vi "Periodic Tasks.vi"(8 "error in (no error)":errorcluster) -> ()   [LabVIEW 2014]
doc: "This VI runs in parallel to other tasks. It can contain as many user-defined periodic loops as you need. These can carry out PID or other sorts of timed response."
uses:
  <vilib>/Rock Robotics/WPI/Joystick/WPI_JoystickGetSetRefNum.vi
  <vilib>/Rock Robotics/WPI/RobotDrive/WPI_RobotDriveGetSetRefNum.vi
panel:
  in  "InputSelect":enum16{"RGB", "ColorBox"}(ring)=enum."ColorBox"
  in  "Position Speed":u32(slide)=20 scale=0.0..200.0
  out "B":u8
  out "G":u8=200
  out "R":u8=39
  out "Resolved Color":u32=2607104 format="%.0x"
  in  "Color Box":u32(colorbox)=12451697
  in  "LED Position":u8(slide)=7 scale=0.0..30.0
  in  "Brightness":u8(slide)=255 scale=0.0..255.0
  out "error out":errorcluster
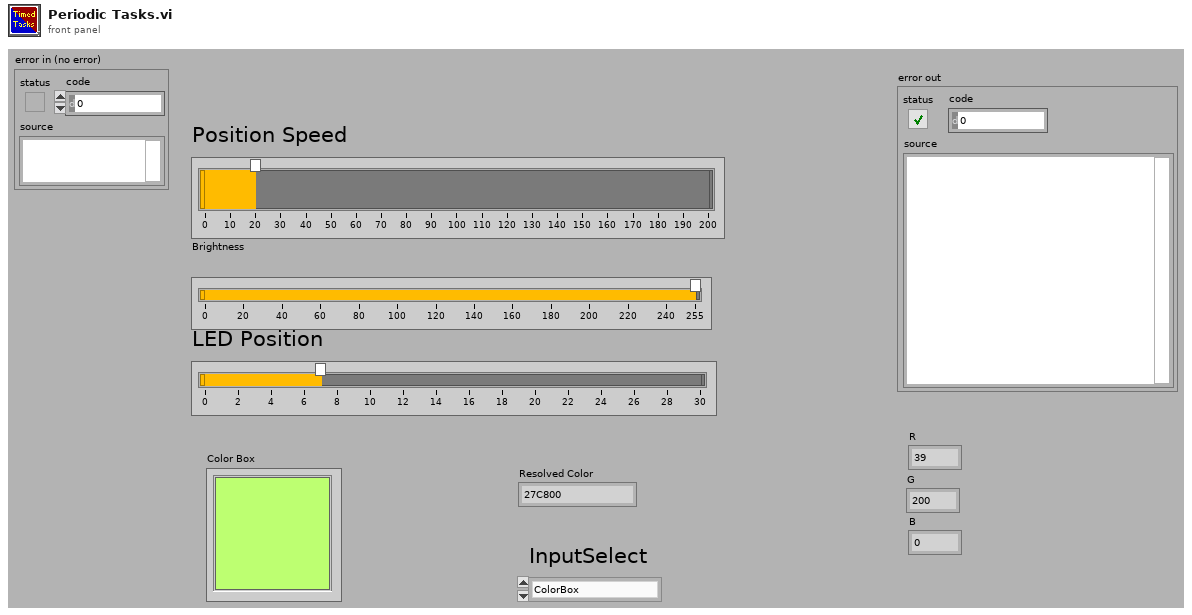
[diagram p1: front panel]
types:
  T1 = typedef "WPI_JoystickDevRef.ctl" = cluster{"Device":T2}
  T2 = typedef "WPI_JoystickDeviceEnum.ctl" = enum16{"USB 0", "USB 1", "USB 2", "USB 3", "USB 4", "USB 5"}
  T3 = typedef "WPI_RobotDriveDevRef.ctl" = cluster{"DevStatus":errorcluster, "Motors[]":T4[], "Square Inputs":bool, "Max Output":dbl}
  T4 = typedef "WPI_MotorControlDeviceRef.ctl" = cluster{"DeviceStatus":errorcluster, "Type":T5, "PWM":cluster{"Controller":T6, "PWM Channel":T7, "DeadBand":T8}, "CAN":cluster{"Device Number":u8, "Control Mode":T9, "Semaphore":T10, "Max Vout":dbl, "TalonSRX Control Mode":T11}, "Invert":bool, "TransformRef":T12, "InvTransformRef":T12}
  T5 = typedef "WPI_MotorControlType.ctl" = enum16{"PWM", "CAN", "CANTalonSRX"}
  T6 = typedef "FPGA_TypedefDigitalModule.ctl" = enum16{"Controller 1"}
  T7 = typedef "FPGA_DIOPWMChannel.ctl" = enum8{"PWM 0", "PWM 1", "PWM 2", "PWM 3", "PWM 4", "PWM 5", "PWM 6", "PWM 7", "PWM 8", "PWM 9", "PWM MXP 0", "PWM MXP 1", "PWM MXP 2", "PWM MXP 3", "PWM MXP 4", "PWM MXP 5", "PWM MXP 6", "PWM MXP 7", "PWM MXP 8", "PWM MXP 9", "Invalid"}
  T8 = typedef "WPI_PWMDeadband.ctl" = cluster{"Name":string, "maxPositivePwm":i32, "minPositivePwm":i32, "centerPwm":i32, "maxNegativePwm":i32, "minNegativePwm":i32, "angularRange":u16}
  T9 = typedef "WPI_CANJaguar_ControlMode.ctl" = enum8{"Percent VBus", "Current", "Speed", "Position", "Voltage"}
  T10 = typedef "Semaphore RefNum" = refnum<k1>
  T11 = typedef "WPI_CANTalonSRX_APIControlMode.ctl" = enum8{"Percent VBus", "Speed", "Position", "Slave", "Unchanged / Invalid"}
  T12 = typedef "WPI_PWMTransform_ConPane.ctl" = refnum<vi>
  T13 = cluster{"JoystickDevRef":T1, "RobotDriveDevRef":T3}
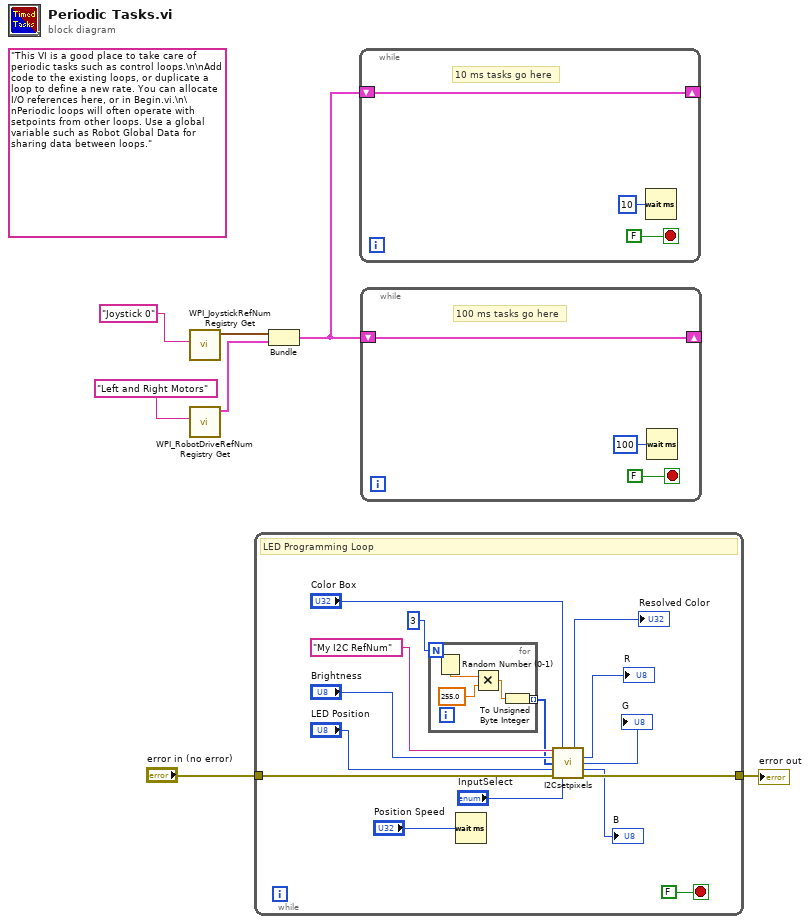
[diagram p0: block diagram]
diagram:
  (unwired) "This VI is a good place to take care of periodic tasks such as control loops.\n\nAdd code to the existing loops, or duplicate a loop to define a new rate. You can allocate I/O references here, or in Begin.vi.\n\nPeriodic loops will often operate with setpoints from other loops. Use a global variable such as Robot Global Data for sharing data between loops."
  n1 = call <vilib>:"WPI_JoystickRefNum Registry Get.vi"("refnum name"="Joystick 0") -> ("JoystickDevRef"=w5:T1)  [unwired: 1 in, 9 out]
  n2 = call <vilib>:"WPI_RobotDriveRefNum Registry Get.vi"("refnum name"="Left and Right Motors") -> ("RobotDriveDevRef"=w4:T3)  [unwired: 1 in, 9 out]
  n3 = while {
    tunnel: "error in (no error)" -> [w21]
    tunnel: [w20] -> w1
    stop <- FALSE stop-if-true
    # "LED Programming Loop"
    n4 = for {
      N: 3 -> [_]
      tunnel: [w23] -> w9 mode=indexing
      n5 = Random Number (0-1)() -> (number: 0 to 1=w25:dbl)
      n6 = Multiply(x=w25, y=255.0) -> (x*y=w24:dbl)
      n7 = To Unsigned Byte Integer(number=w24) -> (unsigned 8bit integer=w23:u8)
    }
    n8 = Wait (ms)(milliseconds to wait="Position Speed") -> ()  [unwired: 1 out]
    n9 = call "I2Csetpixels.vi"("I2C Reference In"="My I2C RefNum" ("refnum name"), "Color Box"="Color Box", "Brightness (0-255)"="Brightness", "RGB Array"=w9, "LED Position"="LED Position", "Error In"=w21, "InputSelect"="InputSelect") -> ("Resolved Color"=→"Resolved Color":u32, "R"=→"R":u8, "G"=→"G":u8, "B"=→"B":u8, "Error Out"=w20:errorcluster)  [unwired: 3 in, 1 out]
  }
  "error out" <- w1
  n10 = Bundle("JoystickDevRef"=w5, "RobotDriveDevRef"=w4) -> (w3:T13)  [unwired: 1 out]
  n11 = while {
    shift-right: [w27] -> _
    shift-left: w3 -> [w27]
    stop <- FALSE stop-if-true
    # "10 ms tasks go here"
    n12 = Wait (ms)(milliseconds to wait=u32 10) -> ()  [unwired: 1 out]
  }
  n13 = while {
    shift-right: [w30] -> _
    shift-left: w3 -> [w30]
    stop <- FALSE stop-if-true
    # "100 ms tasks go here"
    n14 = Wait (ms)(milliseconds to wait=u32 100) -> ()  [unwired: 1 out]
  }
